vi "Waveform - Get Y Value.vi"() -> ()   [LabVIEW 2020]
doc: "Shows how to use the Get Y Value VI from the waveforms operations menu."
uses:
  <vilib>/Waveform/WDTOps.llb/WDT Get XY Value DBL.vi
panel:
  out "Value at Index":dbl
  in  "Index":dbl=10.0
  out "Waveform":waveform(dbl)[](graph)
  # "Overview: Demonstrates how to retrieve the value at a specified index from a waveform with the Get XY Value VI.\nInstructions:\n1. Select an Index value.\n2. Run the VI. The waveform value at the specified Index will be displayed in the Waveform graph."
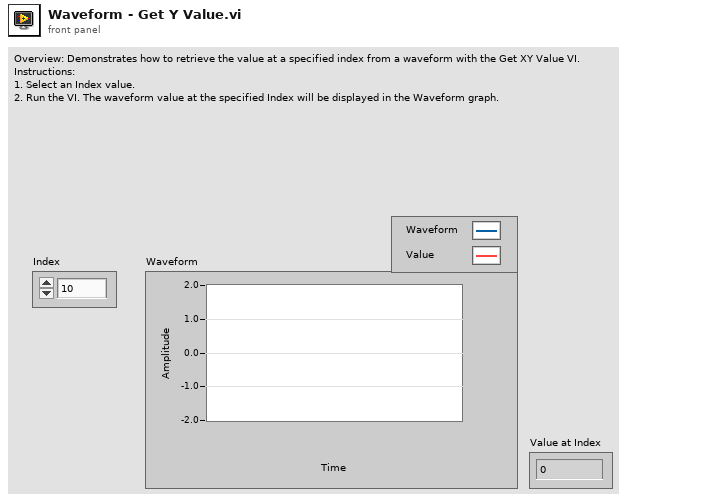
[diagram p1: front panel]
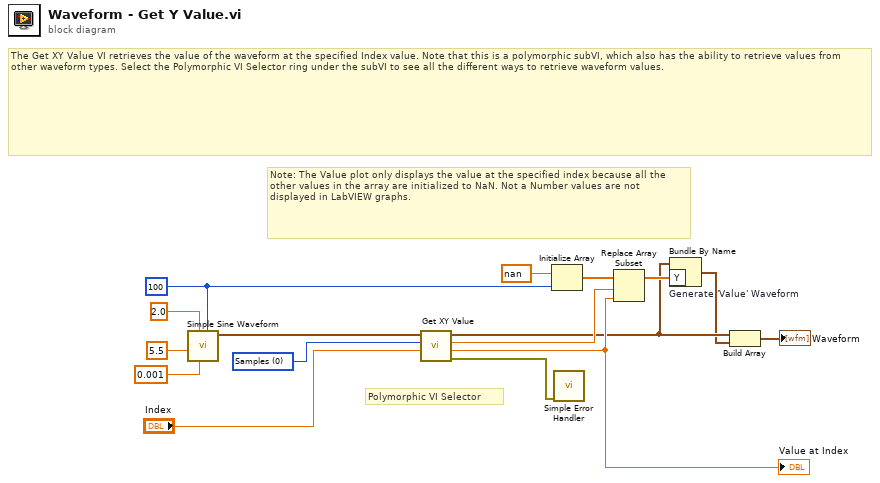
[diagram p0: block diagram]
diagram:
  w2 = u16 0 items=["Samples", "Relative Time"] ("Y position format")
  w4 = 100 ("n points")
  # "The Get XY Value VI retrieves the value of the waveform at the specified Index value. Note that this is a polymorphic subVI, which also has the ability to retrieve values from other waveform types. Select the Polymorphic VI Selector ring under the subVI to see all the different ways to retrieve waveform values."
  # "Polymorphic VI Selector"
  # "Note: The Value plot only displays the value at the specified index because all the other values in the array are initialized to NaN. Not a Number values are not displayed in LabVIEW graphs."
  n1 = call "Simple Sine Waveform.vi"("n points"=w4, "delta t"=0.001, "amplitude"=2.0, "n cycles"=5.5 ("frequency")) -> ("sine waveform"=w15:waveform(dbl))  [unwired: 7 in]
  n2 = call-poly <vilib>:"Get XY Value.vi"("Y position"="Index", "Y position format"=w2, "waveform in"=w15) -> ("error out"=w1:errorcluster, "Y value"=w7:dbl, "actual Y position"=w8:dbl, "waveform out"=w6:waveform(dbl))  [unwired: 4 in, 1 out]
  "Value at Index" <- w7
  n3 = Initialize Array(nan, w4) -> (w9:dbl[])
  n4 = call <vilib>:"Simple Error Handler.vi"("error in (no error)"=w1) -> ()  [unwired: 4 in, 5 out]
  n5 = Replace Array Subset(array=w9, new element=w7, index=w8) -> (w11:dbl[])
  n6 = Bundle By Name "Generate 'Value' Waveform"(cluster=w6, "Y"=w11) -> (w5:waveform(dbl))
  n7 = Build Array(w6, w5) -> (→"Waveform":waveform(dbl)[])
